vi "Magnetic Sweep 1.9b.vi"() -> ()   [LabVIEW 2011]
panel:
  in  "Save":bool
  out "Cryocon end of loop":errorcluster
  out "file position4":errorcluster
  out "file position3":errorcluster
  out "file position2":errorcluster
  out "File position1":errorcluster
  out "Initial Temperature check":errorcluster
  out "Status":i32
  out "Loop end check":errorcluster
  out "Parameter setup":errorcluster
  out "Resistance check":errorcluster
  out "Start ramping":errorcluster
  out "Cell temperature\ncheck":errorcluster
  out "Initial Temp\nCheck":errorcluster
  out "Current time":timestamp format="%<%I:%M:%S %p\n%x>T"
  out "x .and. y?":bool
  in  "Initial\nTemperature":dbl
  out "Heater":bool
  out "Persistent switch ready":bool
  out "Initial check":errorcluster
  in  "Temperature\nlower limite":dbl
  out "Ramping rate command":string
  out "Target field command":string
  out "String":string="Persistent switch is not on"
  in  "Set parameter":bool
  out "status":string
  out "PID command":string
  out "setpoint command":string
  out "setpoint":dbl
  in  "stop":bool
  in  "Contour plot (ramp down)":path
  in  "Raw data (ramp down)":path
  out "Elapsed Time (s)":dbl
  out "Iteration":i32
  out "Zero field reached":bool
  out "Target field reached":bool
  in  "Temperature\nupper limite":dbl
  in  "Temperature\nramping step":dbl
  in  "Heater range":i16(ring) items=["High", "Medium", "Low"]
  in  "D gain":dbl
  in  "I gain":dbl
  in  "P gain":dbl
  in  "Contour plot (ramp up)":path
  in  "Timer":bool caption="Reset"
  in  "Raw data (ramp  up)":path
  out "Current Resistance":string
  out "Current Temperature":string
  out "Current Field":string
  in  "Sweep":bool
  in  "Magnetic field\nRamp rate":dbl
  in  "Traget Field":dbl
  out "Init Response":string
  in  "Update":bool
  in  "P Switch on/off\nafter measurement":bool
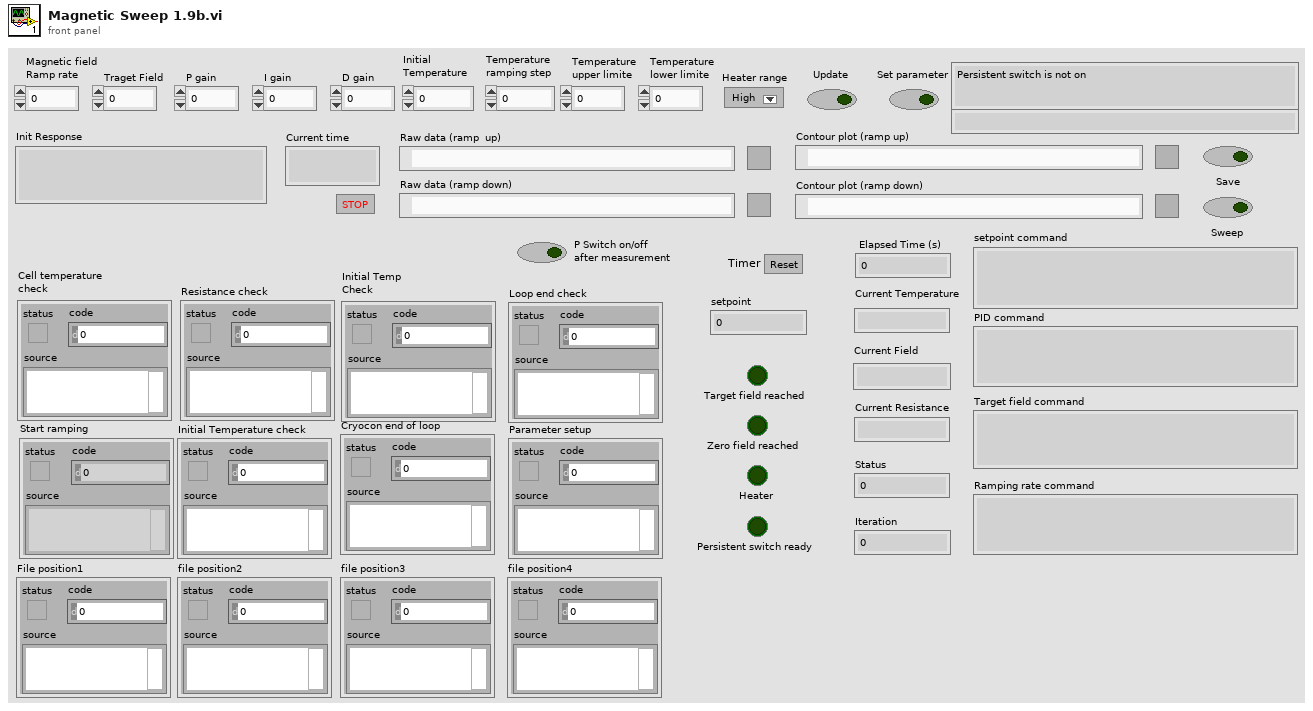
[diagram p1: front panel]
types:
  T1 = enum16{"open", "replace", "create", "open or create", "replace or create", "replace or create with confirmation"}
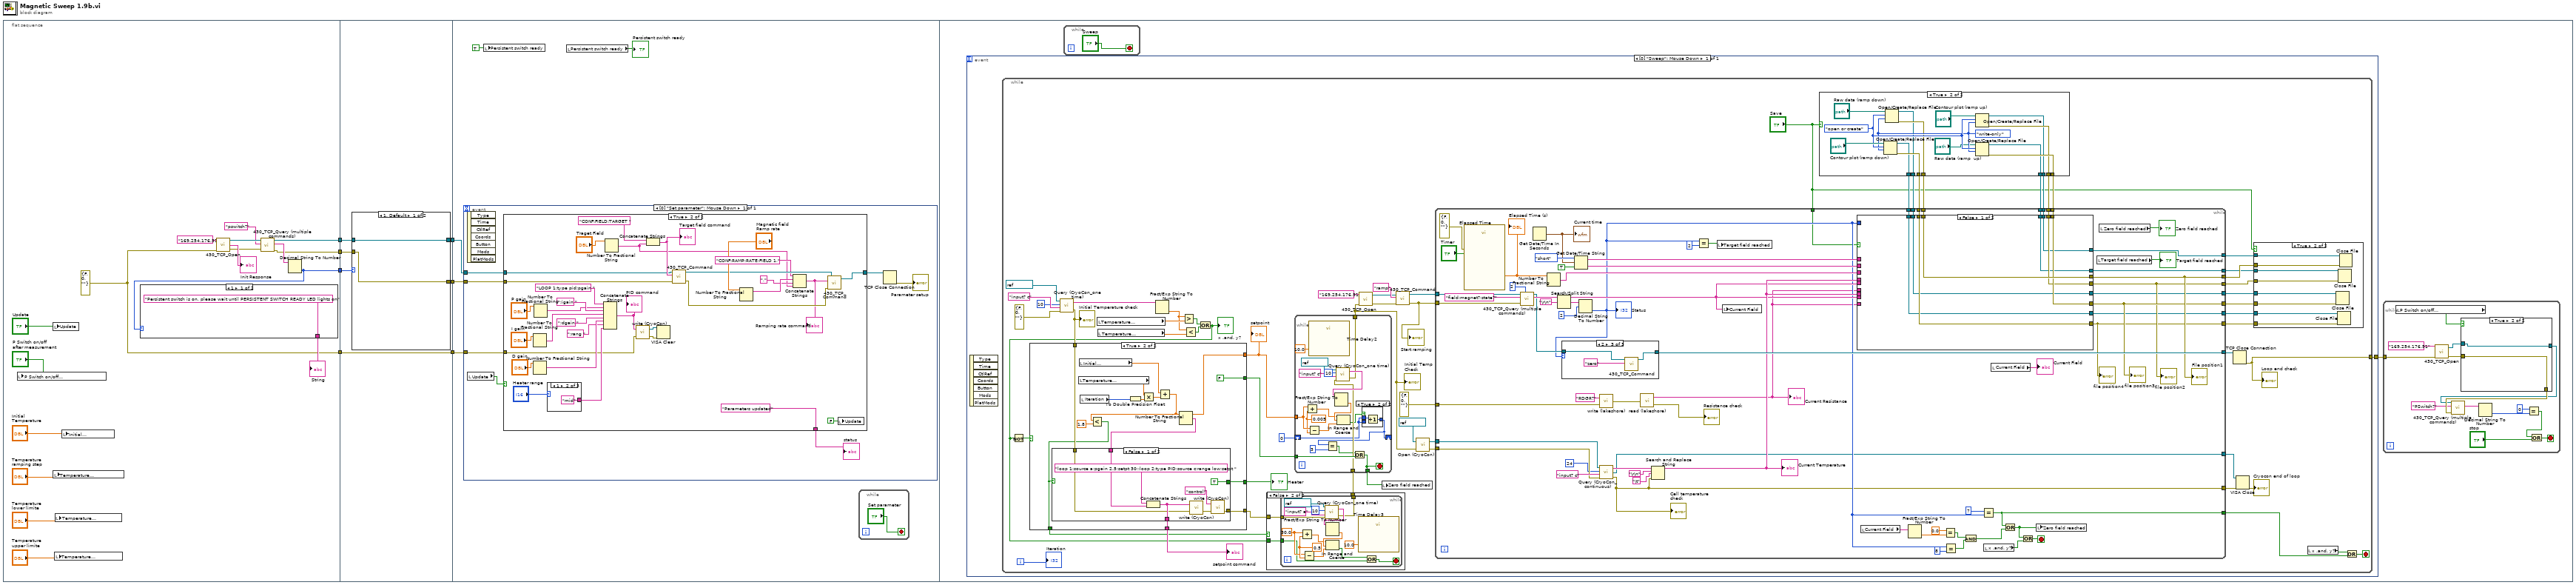
[diagram p0: block diagram]
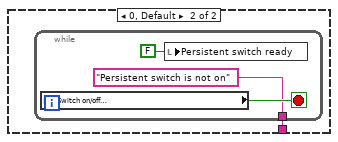
[diagram p2: hidden frame]
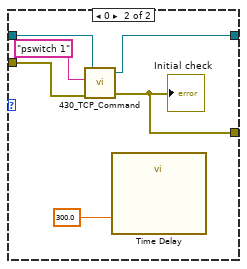
[diagram p3: hidden frame]
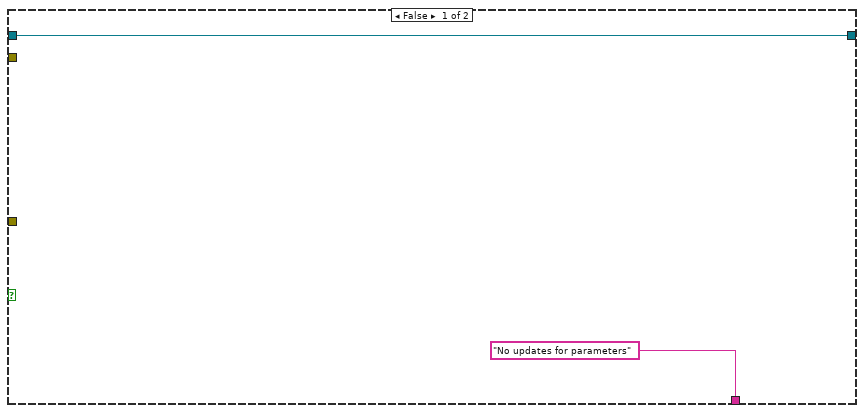
[diagram p4: hidden frame]
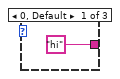
[diagram p5: hidden frame]
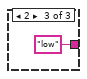
[diagram p6: hidden frame]
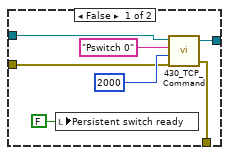
[diagram p7: hidden frame]
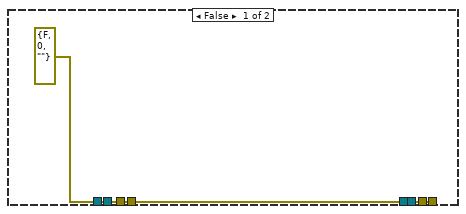
[diagram p9: hidden frame]
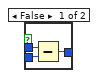
[diagram p11: hidden frame]
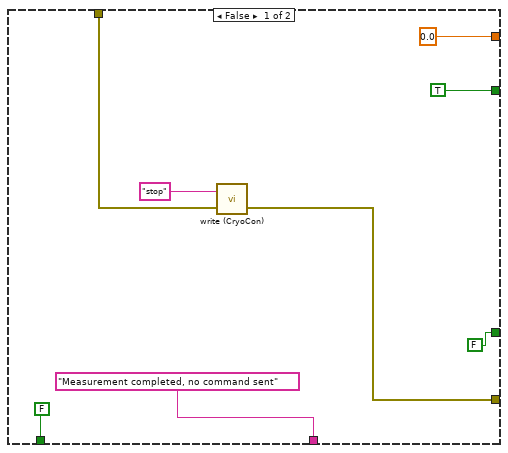
[diagram p12: hidden frame]
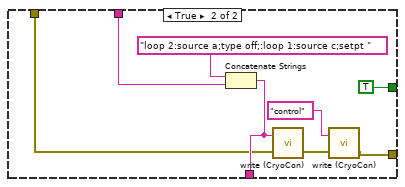
[diagram p13: hidden frame]
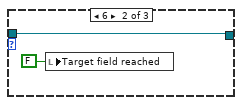
[diagram p15: hidden frame]
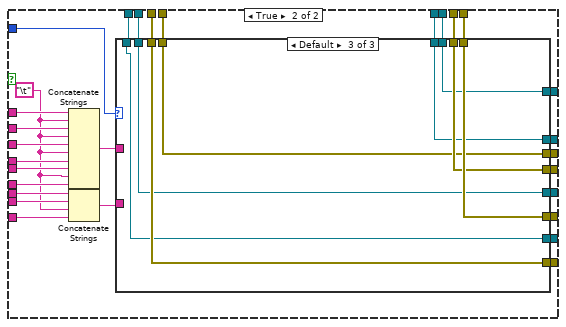
[diagram p16: hidden frame]
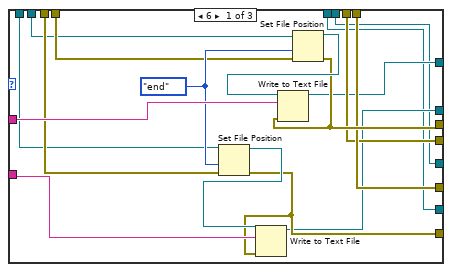
[diagram p17: hidden frame]
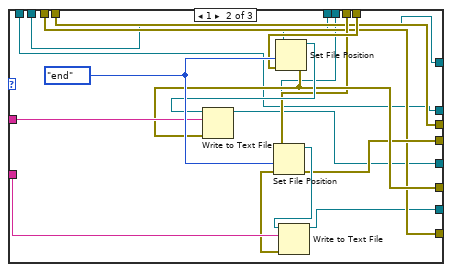
[diagram p18: hidden frame]
diagram:
  n1 = flat-sequence {
    tunnel: [w13] -> w7
    tunnel: [w12] -> w5
    tunnel: [w10] -> w4
    tunnel: [w8] -> w1
    tunnel: w7 -> [w35]
    tunnel: [w34] -> w6
    tunnel: w5 -> [w33]
    tunnel: w4 -> [w32]
    tunnel: [w31] -> w3
    tunnel: [w30] -> w2
    tunnel: w1 -> [w30]
    tunnel: w6 -> [w46]
    tunnel: w3 -> [w45]
    tunnel: w2 -> [w44]
    frame #0 {
      w8 = errorcluster {"status"=FALSE, "code"=0, "source"=""} ("error in (no error)")
      n2 = local write "P Switch on/off\nafter measurement"("P Switch on/off\nafter measurement") -> ()
      n3 = local write "Update"("Update") -> ()
      n4 = local write "Temperature\nramping step"("Temperature\nramping step") -> ()
      n5 = local write "Temperature\nupper limite"("Temperature\nupper limite") -> ()
      n6 = local write "Temperature\nlower limite"("Temperature\nlower limite") -> ()
      n7 = local write "Initial\nTemperature"("Initial\nTemperature") -> ()
      n8 = call "430_TCP_Open.vi"("IP Address"="169.254.176.91", "error in (no error)"=w8) -> ("connection ID"=w19:refnum<k5>, "Init Response"=→"Init Response":string, "error out"=w18:errorcluster)  [unwired: 4 in]
      n9 = call "430_TCP_Query (multiple commands).vi"("error in (no error)"=w18, "Command"="pswitch?", "connection ID"=w19) -> ("error out"=w10:errorcluster, "Response"=w16:string, "connection ID out"=w13:refnum<k5>)  [unwired: 4 in, 2 out]
      n10 = Decimal String To Number(string=w16) -> (number=w12:i32)  [unwired: 2 in, 1 out]
      n11 = case shown="1" w12 {
        tunnel: ["Persistent switch is on, please wait until PERSISTENT SWITCH READY LED lights on" w26] -> w15
        frame 1 {
        }
        frame 0, Default {
          n12 = while {
            tunnel: ["Persistent switch is not on"] -> w26
            stop <- w29 stop-if-true
            n13 = local read "P Switch on/off\nafter measurement"() -> (w29:bool)
            n14 = local write "Persistent switch ready"(FALSE ("Persistent switch ready")) -> ()
          }
        }
      }
      "String" <- w15
    }
    frame #1 {
      n15 = case shown="1, Default" w33 {
        tunnel: w35 -> [w37 w43]
        tunnel: [w37 w42] -> w34
        tunnel: w32 -> [w36 w39]
        tunnel: [w36 w38] -> w31
        frame 1, Default {
        }
        frame 0 {
          n16 = call "430_TCP_Command.vi"("error in (no error)"=w39, "Command"="pswitch 1", "connection ID"=w43) -> ("error out"=w38:errorcluster, "connection ID out"=w42:refnum<k5>)  [unwired: 1 in, 1 out]
          "Initial check" <- w38
          n17 = call "Time Delay"("Delay Time (s)"=300.0) -> ()  [unwired: 10 in, 1 out]
        }
      }
    }
    frame #2 {
      n18 = event shown="[0] \"Set parameter\": Mouse Down" {
        selector: _ -> [_]
        dyn-events: _ -> [_]
        timeout: _ -> [_]
        tunnel: w46 -> [w56]
        tunnel: w45 -> [w51]
        tunnel: w44 -> [w50]
        event "Set parameter": Mouse Down {
          n19 = event-data() -> ()  [unwired: 1 in, 7 out]
          n20 = local read "Update"() -> (w54:bool)
          n21 = case shown="True" w54 {
            tunnel: w56 -> [w57 w88]
            tunnel: ["No updates for parameters" ("String") "Parameters updated" ("String")] -> w55
            tunnel: [w57 w63] -> w53
            tunnel: w51 -> [_ w60]
            tunnel: w50 -> [_ w59]
            frame False {
            }
            frame True {
              n22 = Number To Fractional String(number="I gain") -> (F-format string=w71:string)  [unwired: 3 in]
              n23 = Number To Fractional String(number="D gain") -> (F-format string=w69:string)  [unwired: 3 in]
              n24 = Number To Fractional String(number="P gain") -> (F-format string=w72:string)  [unwired: 3 in]
              n25 = case shown="1" "Heater range" {
                tunnel: ["hi" "mid" "low"] -> w65
                frame 0, Default {
                }
                frame 1 {
                }
                frame 2 {
                }
              }
              n26 = Concatenate Strings("LOOP 1:type pid;pgain " ("write buffer"), w72, ";igain " ("string"), w71, ";dgain " ("string"), w69, ";rang " ("string"), w65) -> (w68:string)
              "PID command" <- w68
              n27 = Number To Fractional String(number="Traget Field") -> (F-format string=w78:string)  [unwired: 3 in]
              n28 = call "write (CryoCon).vi"("error in (no error)"=w59, "write buffer"=w68) -> ("error out"=w62:errorcluster, "VISA resource name out"=w61:refnum<visa-resource-name>)
              n29 = Concatenate Strings("CONF:FIELD:TARGET ", w78) -> (w89:string)
              "Target field command" <- w89
              n30 = VISA Clear(VISA resource name=w61, error in (no error)=w62) -> ()  [unwired: 2 out]
              n31 = call "430_TCP_Command.vi"("error in (no error)"=w60, "Command"=w89, "connection ID"=w88) -> ("error out"=w87:errorcluster, "connection ID out"=w83:refnum<k5>)  [unwired: 1 in, 1 out]
              n32 = Number To Fractional String(number="Magnetic field\nRamp rate") -> (F-format string=w81:string)  [unwired: 3 in]
              n33 = Concatenate Strings("CONF:RAMP:RATE:FIELD 1," ("string"), w81, "," ("string"), w78) -> (w84:string)
              "Ramping rate command" <- w84
              n34 = call "430_TCP_Command.vi"("error in (no error)"=w87, "Command"=w84, "connection ID"=w83) -> ("connection ID out"=w63:refnum<k5>)  [unwired: 1 in, 2 out]
              n35 = local write "Update"(FALSE ("Update")) -> ()
            }
          }
          "status" <- w55
          n36 = TCP Close Connection(connection ID=w53) -> (error out=→"Parameter setup":errorcluster)  [unwired: 2 in, 1 out]
        }
      }
      n37 = local write "Persistent switch ready"(TRUE ("Persistent switch ready")) -> ()
      n38 = local read "Persistent switch ready"() -> (→"Persistent switch ready":bool)
      n39 = while {
        stop <- "Set parameter" stop-if-true
      }
    }
    frame #3 {
      n40 = event shown="[0] \"Sweep\": Mouse Down" {
        selector: _ -> [_]
        dyn-events: _ -> [_]
        timeout: _ -> [_]
        tunnel: [w119] -> w94
        event "Sweep": Mouse Down {
          n41 = event-data() -> ()  [unwired: 1 in, 7 out]
          n42 = while {
            tunnel: [w149] -> w119
            i -> [w177]
            stop <- w164 stop-if-true
            n43 = call "Query (CryoCon_one time).vi"("error in (no error)"=errorcluster {"status"=FALSE, "code"=0, "source"=""}, "write buffer"="input? c", "byte count"=u32 10, "VISA resource name 2"=refnum<visa-resource-name> "COM3") -> ("error out"=w162:errorcluster, "read buffer"=w173:string)
            "Initial Temperature check" <- w162
            n44 = local read "Temperature\nupper limite"() -> (w175:dbl)
            n45 = local read "Temperature\nlower limite"() -> (w170:dbl)
            n46 = Fract/Exp String To Number(string=w173) -> (number=w171:dbl)  [unwired: 3 in, 1 out]
            n47 = Greater?(x=w171, y=w175) -> (0:w168:bool)
            n48 = Less?(x=w171, y=w170) -> (x < y?=w169:bool)
            n49 = Or(x=w168, y=w169) -> (x .or. y?=w154:bool)
            "x .and. y?" <- w154
            n50 = Not(x=w154) -> (.not. x?=w161:bool)
            n51 = case shown="True" w161 {
              tunnel: [w246 w261] -> w156
              tunnel: [0.0 w259] -> w178
              tunnel: ["Measurement completed, no command sent" w262] -> w160
              tunnel: [TRUE FALSE] -> w167
              tunnel: w162 -> [w248 w255]
              tunnel: [FALSE ("Heater") w254] -> w158
              tunnel: [FALSE w253] -> w157
              frame False {
                n52 = call "write (CryoCon).vi"("error in (no error)"=w248, "write buffer"="stop") -> ("error out"=w246:errorcluster)  [unwired: 1 out]
              }
              frame True {
                n53 = local read "Temperature\nramping step"() -> (w264:dbl)
                n54 = local read "Initial\nTemperature"() -> (w257:dbl)
                n55 = local read "Iteration"() -> (w256:i32)
                n56 = To Double Precision Float(number=w256) -> (double precision float=w263:dbl)
                n57 = Multiply(x=w264, y=w263) -> (x*y=w265:dbl)
                n58 = Add(x=w257, y=w265) -> (x+y=w259:dbl)
                n59 = Less?(x=w259, y=1.8) -> (x < y?=w253:bool)
                n60 = Number To Fractional String(number=w259) -> (F-format string=w266:string)  [unwired: 3 in]
                n61 = case shown="False" w253 {
                  tunnel: w266 -> [w273 w281]
                  tunnel: [w270 w280] -> w262
                  tunnel: [w272 w279] -> w261
                  tunnel: w255 -> [w267 w276]
                  tunnel: [TRUE ("Heater") TRUE ("Heater")] -> w254
                  frame False {
                    n62 = Concatenate Strings("loop 1:source a;pgain 2.5;setpt 30;:loop 2:type PID;source c;range low;setpt " ("write buffer"), w273) -> (w270:string)
                    n63 = call "write (CryoCon).vi"("error in (no error)"=w267, "write buffer"=w270) -> ("error out"=w269:errorcluster)  [unwired: 1 out]
                    n64 = call "write (CryoCon).vi"("error in (no error)"=w269, "write buffer"="control") -> ("error out"=w272:errorcluster)  [unwired: 1 out]
                  }
                  frame True {
                    n65 = Concatenate Strings("loop 2:source a;type off;:loop 1:source c;setpt " ("write buffer"), w281) -> (w280:string)
                    n66 = call "write (CryoCon).vi"("error in (no error)"=w276, "write buffer"=w280) -> ("error out"=w278:errorcluster)  [unwired: 1 out]
                    n67 = call "write (CryoCon).vi"("error in (no error)"=w278, "write buffer"="control") -> ("error out"=w279:errorcluster)  [unwired: 1 out]
                  }
                }
              }
            }
            "setpoint" <- w178
            "setpoint command" <- w160
            "Heater" <- w158
            n68 = case shown="False" w157 {
              tunnel: w156 -> [w202 w205]
              tunnel: [w202 w203] -> w155
              tunnel: w154 -> [_ w204]
              frame True {
              }
              frame False {
                n69 = while {
                  tunnel: w205 -> [w217]
                  tunnel: w204 -> [w209]
                  tunnel: [w207] -> w203
                  stop <- w208 stop-if-true
                  w211 = 30.0 ("x")
                  w212 = 0.5 ("y")
                  n70 = Add(x=w211, y=w212) -> (x+y=w214:dbl)
                  n71 = Subtract(x=w211, y=w212) -> (x-y=w213:dbl)
                  n72 = call "Query (CryoCon_one time).vi"("error in (no error)"=w217, "write buffer"="input? a", "byte count"=u32 10, "VISA resource name 2"=refnum<visa-resource-name> "COM3") -> ("error out"=w207:errorcluster, "read buffer"=w216:string)
                  n73 = Fract/Exp String To Number(string=w216) -> (number=w215:dbl)  [unwired: 3 in, 1 out]
                  n74 = In Range and Coerce(upper limit=w214, x=w215, lower limit=w213) -> (In Range?=w210:bool)  [unwired: 1 out]
                  n75 = call "Time Delay3"("Delay Time (s)"=10.0) -> ()  [unwired: 10 in, 1 out]
                  n76 = Or(x=w210, y=w209) -> (x .or. y?=w208:bool)
                }
              }
            }
            n77 = while {
              tunnel: w178 -> [w238]
              tunnel: w167 -> [w230]
              tunnel: [w229] -> w137
              tunnel: [w228] -> w159
              tunnel: w155 -> [w227]
              shift-right: [w225] -> _
              shift-left: 0 -> [w222]
              stop <- w228 stop-if-true
              w235 = 0.005 ("y")
              n78 = Add(x=w238, y=w235) -> (x+y=w237:dbl)
              n79 = Subtract(x=w238, y=w235) -> (x-y=w236:dbl)
              n80 = call "Time Delay2"("Delay Time (s)"=10.0) -> ()  [unwired: 10 in, 1 out]
              n81 = call "Query (CryoCon_one time).vi"("error in (no error)"=w227, "write buffer"="input? c", "byte count"=u32 10, "VISA resource name 2"=refnum<visa-resource-name> "COM3") -> ("error out"=w229:errorcluster, "read buffer"=w232:string)
              n82 = Fract/Exp String To Number(string=w232) -> (number=w239:dbl)  [unwired: 3 in, 1 out]
              n83 = In Range and Coerce(upper limit=w237, x=w239, lower limit=w236) -> (In Range?=w226:bool)  [unwired: 1 out]
              n84 = case shown="True" w226 {
                tunnel: w222 -> [w242 w243]
                tunnel: [w240 w244] -> w225
                tunnel: w222 -> [w241 _]
                frame False {
                  n85 = Subtract(x=w242, y=w241) -> (x-y=w240:i32)
                }
                frame True {
                  n86 = Increment(x=w243) -> (x+1=w244:i32)
                }
              }
              n87 = Equal?(x=w225, y=3) -> (x = y?=w224:bool)
              n88 = Or(x=w224, y=w230) -> (x .or. y?=w228:bool)
            }
            "Initial Temp\nCheck" <- w137
            n89 = call "430_TCP_Open.vi"("IP Address"="169.254.176.91", "error in (no error)"=w137) -> ("connection ID"=w152:refnum<k5>, "error out"=w153:errorcluster)  [unwired: 4 in, 1 out]
            n90 = local write "Zero field reached"(w159) -> ()
            n91 = call "430_TCP_Command.vi"("error in (no error)"=w153, "Command"="ramp", "connection ID"=w152) -> ("error out"=w151:errorcluster, "connection ID out"=w166:refnum<k5>)  [unwired: 1 in, 1 out]
            "Start ramping" <- w151
            n92 = call "Open (CryoCon).vi"("error in (no error)"=w137, "VISA resource name"=refnum<visa-resource-name> "COM3") -> ("error out"=w143:errorcluster, "VISA resource name out"=w144:refnum<visa-resource-name>)
            n93 = case shown="True" "Save" {
              tunnel: [w187 w195] -> w134
              tunnel: [w187 w194] -> w133
              tunnel: [w187 w193] -> w136
              tunnel: [w187 w192] -> w135
              tunnel: [_ w191] -> w128
              tunnel: [_ w190] -> w127
              tunnel: [_ w189] -> w126
              tunnel: [_ w188] -> w125
              frame False {
                w187 = errorcluster {"status"=FALSE, "code"=0, "source"=""} ("error out")
              }
              frame True {
                w198 = enum16{"read/write", "read-only", "write-only"}."write-only" ("access (0:read/write)")
                w199 = T1."open or create" ("operation (0:open)")
                n94 = Open/Create/Replace File(file path (use dialog)="Contour plot (ramp down)", operation (0:open)=w199, access (0:read/write)=w198) -> (refnum out=w190:refnum<file>, error out=w194:errorcluster)  [unwired: 3 in, 1 out]
                n95 = Open/Create/Replace File(file path (use dialog)="Raw data (ramp down)", operation (0:open)=w199, access (0:read/write)=w198) -> (refnum out=w191:refnum<file>, error out=w195:errorcluster)  [unwired: 3 in, 1 out]
                n96 = Open/Create/Replace File(file path (use dialog)="Contour plot (ramp up)", operation (0:open)=w199, access (0:read/write)=w198) -> (refnum out=w188:refnum<file>, error out=w192:errorcluster)  [unwired: 3 in, 1 out]
                n97 = Open/Create/Replace File(file path (use dialog)="Raw data (ramp  up)", operation (0:open)=w199, access (0:read/write)=w198) -> (refnum out=w189:refnum<file>, error out=w193:errorcluster)  [unwired: 3 in, 1 out]
              }
            }
            n98 = while {
              tunnel: w166 -> [w347]
              tunnel: [w333] -> w165
              tunnel: w151 -> [w327]
              tunnel: [w326] -> w150
              tunnel: w144 -> [w305]
              tunnel: w143 -> [w304]
              tunnel: errorcluster {"status"=FALSE, "code"=0, "source"=""} ("error in (no error)") -> [w303]
              tunnel: [w302] -> w141
              tunnel: [w301] -> w140
              tunnel: w136 -> [w299]
              tunnel: w135 -> [w298]
              tunnel: w134 -> [w297]
              tunnel: w133 -> [w296]
              tunnel: [w295] -> w132
              tunnel: [w287] -> w131
              tunnel: [w294] -> w130
              tunnel: [w288] -> w129
              tunnel: w128 -> [w293]
              tunnel: w127 -> [w292]
              tunnel: w126 -> [w291]
              tunnel: w125 -> [w290]
              tunnel: "Save" -> [w289]
              tunnel: [w286] -> w123
              tunnel: [w285] -> w122
              tunnel: [w284] -> w121
              tunnel: [w283] -> w120
              stop <- w335 stop-if-true
              n99 = call "Elapsed Time"("Reset"="Timer", "error in (no error)"=errorcluster {"status"=FALSE, "code"=0, "source"=""}) -> ("Elapsed Time (s)"=w345:dbl)  [unwired: 10 in, 7 out]
              "Elapsed Time (s)" <- w345
              n100 = call "430_TCP_Query (multiple commands).vi"("Number of\nquerys"=2 ("Number of\nquerys"), "error in (no error)"=w327, "Command"="field:magnet?;state?", "connection ID"=w347) -> ("Response"=w316:string, "connection ID out"=w314:refnum<k5>)  [unwired: 3 in, 3 out]
              n101 = Get Date/Time In Seconds() -> (seconds since 1Jan1904=w324:timestamp)
              "Current time" <- w324
              n102 = Number To Fractional String(number=w345) -> (F-format string=w319:string)  [unwired: 3 in]
              n103 = Search/Split String(string=w316, search string/char (-)="\r\n") -> (substring before match=w313:string, match + rest of string=w309:string)  [unwired: 1 in, 1 out]
              n104 = Get Date/Time String(date format (0)=enum16{"short", "long", "abbreviated"}."short", seconds (now)=w324, want seconds? (F)=TRUE) -> (date string=w321:string, time string=w320:string)
              n105 = Decimal String To Number(string=w309, offset=2) -> (number=w308:i32)  [unwired: 1 in, 1 out]
              "Status" <- w308
              n106 = case shown="2" w308 {
                tunnel: [w353 w354 w357] -> w326
                tunnel: w314 -> [w353 w354 w356]
                frame 0, Default {
                }
                frame 6 {
                  n107 = local write "Target field reached"(FALSE ("Target field reached")) -> ()
                }
                frame 2 {
                  n108 = call "430_TCP_Command.vi"("Command"="zero", "connection ID"=w356) -> ("connection ID out"=w357:refnum<k5>)  [unwired: 2 in, 2 out]
                }
              }
              n109 = call "write (lakeshore).vi"("error in (no error)"=w303, "write buffer"="RDGR?") -> ("error out"=w351:errorcluster)
              n110 = call "Query (CryoCon_continuous).vi"("error in (no error)"=w304, "write buffer"="input? c", "byte count"=u32 24, "VISA resource name"=w305) -> ("error out"=w302:errorcluster, "VISA resource name out"=w301:refnum<visa-resource-name>, "read buffer"=w312:string)
              "Cell temperature\ncheck" <- w302
              n111 = call "read (lakeshore).vi"("error in (no error)"=w351) -> ("read buffer"=w306:string, "error out"=→"Resistance check":errorcluster)
              "Current Resistance" <- w306
              n112 = Search and Replace String(input string=w312, search string="\r\n", replace string="\t", error in=w302) -> (result string=w318:string)  [unwired: 4 in, 3 out]
              "Current Temperature" <- w318
              n113 = Equal?(x=w308, y=2) -> (x = y?=w346:bool)
              n114 = local write "Target field reached"(w346) -> ()
              n115 = local write "Current Field"(w313) -> ()
              n116 = case shown="False" w289 {
                tunnel: w308 -> [_ w395]
                tunnel: w321 -> [_ w392]
                tunnel: w320 -> [_ w391]
                tunnel: w319 -> [_ w390]
                tunnel: w318 -> [_ w389]
                tunnel: w313 -> [_ w388]
                tunnel: w306 -> [_ w381]
                tunnel: w318 -> [_ w387]
                tunnel: w313 -> [_ w386]
                tunnel: [w363 w385] -> w288
                tunnel: [w364 w384] -> w294
                tunnel: [w365 w383] -> w287
                tunnel: w306 -> [_ w382]
                tunnel: w299 -> [w364 w379]
                tunnel: w298 -> [w363 w378]
                tunnel: w297 -> [w366 w377]
                tunnel: w296 -> [w365 w376]
                tunnel: [w366 w375] -> w295
                tunnel: w293 -> [w360 w374]
                tunnel: w292 -> [w359 w373]
                tunnel: w291 -> [w361 w372]
                tunnel: w290 -> [w362 w371]
                tunnel: [w362 w370] -> w286
                tunnel: [w361 w369] -> w285
                tunnel: [w360 w368] -> w284
                tunnel: [w359 w367] -> w283
                frame False {
                }
                frame True {
                  w380 = "\t"
                  n117 = Concatenate Strings(w392, w380, w391, w380, w390, w380, w389, w388, w380, w381) -> (w394:string)
                  n118 = Concatenate Strings(w387, w386, w380, w382) -> (w393:string)
                  n119 = case shown="Default" w395 {
                    tunnel: w394 -> [w412 w428 _]
                    tunnel: w393 -> [w411 w427 _]
                    tunnel: [w402 w423 w436] -> w385
                    tunnel: [w403 w424 w437] -> w384
                    tunnel: [w407 w420 w434] -> w383
                    tunnel: w379 -> [w403 w422 w437]
                    tunnel: w378 -> [w402 w421 w436]
                    tunnel: w377 -> [w406 w419 w435]
                    tunnel: w376 -> [w405 w420 w434]
                    tunnel: [w404 w419 w435] -> w375
                    tunnel: w374 -> [w401 w414 w431]
                    tunnel: w373 -> [w400 w413 w430]
                    tunnel: w372 -> [w396 w418 w432]
                    tunnel: w371 -> [w397 w417 w433]
                    tunnel: [w399 w414 w433] -> w370
                    tunnel: [w398 w413 w432] -> w369
                    tunnel: [w397 w416 w431] -> w368
                    tunnel: [w396 w415 w430] -> w367
                    frame 6 {
                      w410 = enum16{"start", "end", "current"}."end" ("from (0:start)")
                      n120 = Set File Position(refnum=w400, from (0:start)=w410, error in=w405) -> (refnum out=w408:refnum<file>, error out=w407:errorcluster)  [unwired: 1 in]
                      n121 = Write to Text File(file (use dialog)=w408, text=w411, error in=w407) -> (refnum out=w398:refnum<file>)  [unwired: 1 in, 2 out]
                      n122 = Set File Position(refnum=w401, from (0:start)=w410, error in=w406) -> (refnum out=w409:refnum<file>, error out=w404:errorcluster)  [unwired: 1 in]
                      n123 = Write to Text File(file (use dialog)=w409, text=w412, error in=w404) -> (refnum out=w399:refnum<file>)  [unwired: 1 in, 2 out]
                    }
                    frame 1 {
                      w429 = enum16{"start", "end", "current"}."end" ("from (0:start)")
                      n124 = Set File Position(refnum=w417, from (0:start)=w429, error in=w421) -> (refnum out=w425:refnum<file>, error out=w423:errorcluster)  [unwired: 1 in]
                      n125 = Set File Position(refnum=w418, from (0:start)=w429, error in=w422) -> (refnum out=w426:refnum<file>, error out=w424:errorcluster)  [unwired: 1 in]
                      n126 = Write to Text File(file (use dialog)=w426, text=w428, error in=w424) -> (refnum out=w416:refnum<file>)  [unwired: 1 in, 2 out]
                      n127 = Write to Text File(file (use dialog)=w425, text=w427, error in=w423) -> (refnum out=w415:refnum<file>)  [unwired: 1 in, 2 out]
                    }
                    frame Default {
                    }
                  }
                }
              }
              "file position4" <- w287
              "file position3" <- w294
              "file position2" <- w288
              "File position1" <- w295
              n128 = local read "Current Field"() -> (w329:string)
              n129 = Fract/Exp String To Number(string=w329) -> (number=w330:dbl)  [unwired: 3 in, 1 out]
              n130 = Equal?(x=0.0, y=w330) -> (x = y?=w338:bool)
              n131 = Equal?(x=w308, y=8) -> (x = y?=w339:bool)
              n132 = And(x=w338, y=w339) -> (x .and. y?=w337:bool)
              n133 = Equal?(x=7, y=w308) -> (x = y?=w333:bool)
              n134 = local read "x .and. y?"() -> (w334:bool)
              n135 = local read "Current Field"() -> (→"Current Field":string)
              n136 = Or(x=w333, y=w337) -> (x .or. y?=w336:bool)
              n137 = Or(x=w336, y=w334) -> (x .or. y?=w335:bool)
              n138 = local write "Zero field reached"(w336) -> ()
              n139 = local read "Target field reached"() -> (→"Target field reached":bool)
              n140 = local read "Zero field reached"() -> (→"Zero field reached":bool)
            }
            n141 = TCP Close Connection(connection ID=w150) -> (error out=w149:errorcluster)  [unwired: 2 in, 1 out]
            "Loop end check" <- w149
            n142 = VISA Close(VISA resource name=w140, error in (no error)=w141) -> (error out=→"Cryocon end of loop":errorcluster)
            n143 = case shown="True" "Save" {
              tunnel: w132 -> [_ w186]
              tunnel: w131 -> [_ w185]
              tunnel: w130 -> [_ w184]
              tunnel: w129 -> [_ w183]
              tunnel: w123 -> [_ w182]
              tunnel: w122 -> [_ w181]
              tunnel: w121 -> [_ w180]
              tunnel: w120 -> [_ w179]
              frame False {
              }
              frame True {
                n144 = Close File(refnum=w180, error in=w184) -> ()  [unwired: 2 out]
                n145 = Close File(refnum=w179, error in=w185) -> ()  [unwired: 2 out]
                n146 = Close File(refnum=w181, error in=w183) -> ()  [unwired: 2 out]
                n147 = Close File(refnum=w182, error in=w186) -> ()  [unwired: 2 out]
              }
            }
            n148 = local read "x .and. y?"() -> (w163:bool)
            n149 = Or(x=w163, y=w165) -> (x .or. y?=w164:bool)
            "Iteration" <- w177
          }
        }
      }
      n150 = while {
        stop <- "Sweep" stop-if-true
      }
      n151 = while {
        tunnel: w94 -> [w97]
        stop <- w100 stop-if-true
        n152 = local read "P Switch on/off\nafter measurement"() -> (w109:bool)
        n153 = call "430_TCP_Open.vi"("IP Address"="169.254.176.91", "error in (no error)"=w97) -> ("connection ID"=w99:refnum<k5>, "error out"=w98:errorcluster)  [unwired: 4 in, 1 out]
        n154 = case shown="True" w109 {
          tunnel: [w113 w117] -> w107
          tunnel: [w112 w118] -> w106
          tunnel: w99 -> [w111 w118]
          tunnel: w98 -> [w110 w117]
          frame False {
            n155 = local write "Persistent switch ready"(FALSE ("Persistent switch ready")) -> ()
            n156 = call "430_TCP_Command.vi"("error in (no error)"=w110, "Timeout"=2000, "Command"="Pswitch 0", "connection ID"=w111) -> ("error out"=w113:errorcluster, "connection ID out"=w112:refnum<k5>)  [unwired: 1 out]
          }
          frame True {
          }
        }
        n157 = call "430_TCP_Query (multiple commands).vi"("error in (no error)"=w107, "Command"="PSwitch?", "connection ID"=w106) -> ("Response"=w104:string)  [unwired: 4 in, 4 out]
        n158 = Decimal String To Number(string=w104) -> (number=w103:i32)  [unwired: 2 in, 1 out]
        n159 = Equal?(x=0, y=w103) -> (x = y?=w101:bool)
        n160 = Or(x=w101, y="stop") -> (x .or. y?=w100:bool)
      }
    }
  }
